vi "Init.vi"(8 "error in (no error)":errorcluster, 9 "Mode (F=Mul / T = dB)":bool, 10 "Volume":dbl, 11 "Input Name":string) -> (0 "error out":errorcluster, 3 "SetInputVolume out":refnum<class "SetInputVolume.lvclass">)   [LabVIEW 2020, in "obs-websocket.lvlib" / "SetInputVolume.lvclass"]
uses:
  SetInputVolume.lvclass
  SetInputVolume.lvclass/SetInputVolume.ctl
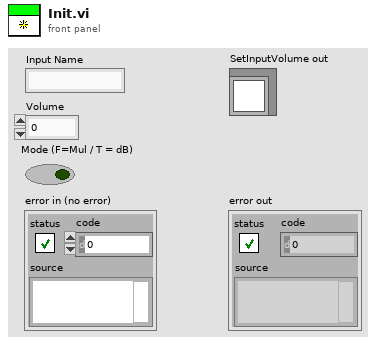
[diagram p1: front panel]
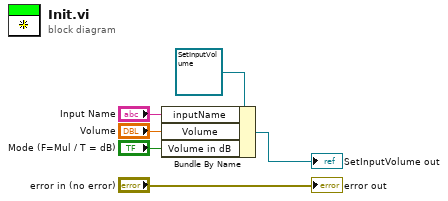
[diagram p0: block diagram]
diagram:
  n1 = Bundle By Name(cluster=refnum<class "SetInputVolume.lvclass"> refnum ("SetInputVolume in"), "inputName"="Input Name", "Volume"="Volume", "Volume in dB"="Mode (F=Mul / T = dB)") -> (→"SetInputVolume out":refnum<class "SetInputVolume.lvclass">)
  "error out" <- "error in (no error)"
